vi "Match Closing Character.vi"(10 "Open character":string, 11 "JSON":string) -> (1 "offset past match":i32, 2 "rest of JSON":string, 3 "match":string)   [LabVIEW 2015, in "NI_Azure_JSON Parsing.lvlib"]
uses:
  NI_Azure_JSON Parsing.lvlib
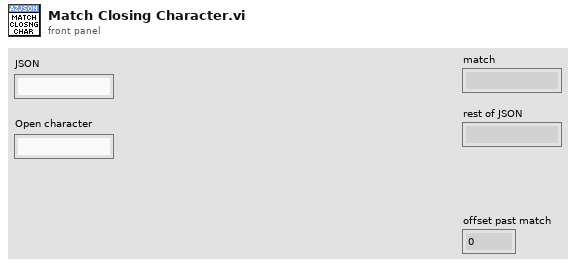
[diagram p1: front panel]
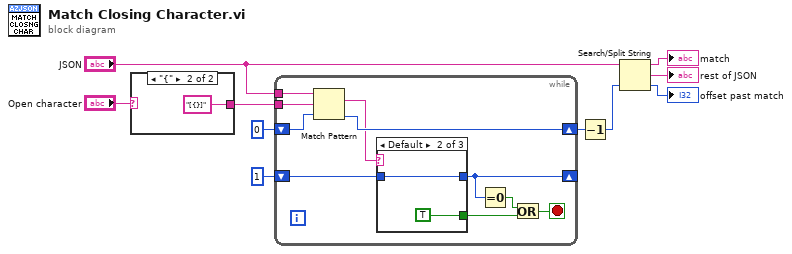
[diagram p0: block diagram]
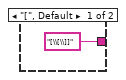
[diagram p2: hidden frame]
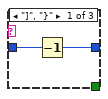
[diagram p3: hidden frame]
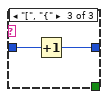
[diagram p4: hidden frame]
diagram:
  n1 = case shown="\"{\"" "Open character" {
    tunnel: ["[\\[\\]]" ("regular expression") "[{}]" ("regular expression")] -> w6
    frame "[", Default {
    }
    frame "{" {
    }
  }
  n2 = while {
    tunnel: "JSON" -> [w20]
    shift-right: [w19] -> w5
    shift-left: 0 -> [w21]
    shift-right: [w16] -> _
    shift-left: 1 -> [w18]
    tunnel: w6 -> [w12]
    stop <- w13 stop-if-true
    n3 = Match Pattern(string=w20, regular expression=w12, offset (0)=w21) -> (match substring=w17:string, offset past match=w19:i32)  [unwired: 2 out]
    n4 = case shown="Default" w17 {
      tunnel: w18 -> [w23 w24 w27]
      tunnel: [_ TRUE _] -> w15
      tunnel: [w22 w24 w26] -> w16
      frame "]", "}" {
        n5 = Decrement(x=w23) -> (x-1=w22:i32)
      }
      frame Default {
      }
      frame "[", "{" {
        n6 = Increment(x=w27) -> (x+1=w26:i32)
      }
    }
    n7 = Equal To 0?(x=w16) -> (x = 0?=w14:bool)
    n8 = Or(x=w14, y=w15) -> (x .or. y?=w13:bool)
  }
  n9 = Decrement(x=w5) -> (x-1=w1:i32)
  "offset past match" <- w1
  n10 = Search/Split String(string="JSON", offset (0)=w1) -> (substring before match=→"match":string, match + rest of string=→"rest of JSON":string)  [unwired: 1 in, 1 out]
